vi "ReadInlineCNode.vi"(2 "reference":refnum<vi>) -> (1 "output cluster":T6)   [LabVIEW 2013]
uses:
  <vilib>/Utility/miscctls.llb/LVBoundsTypeDef.ctl
  <vilib>/Utility/miscctls.llb/LVRectTypeDef.ctl
  <vilib>/Utility/miscctls.llb/LVPositionTypeDef.ctl
  <vilib>/Utility/miscctls.llb/LVBreakpointStatusEnum.ctl
  <vilib>/picture/picture.llb/imagedata.ctl
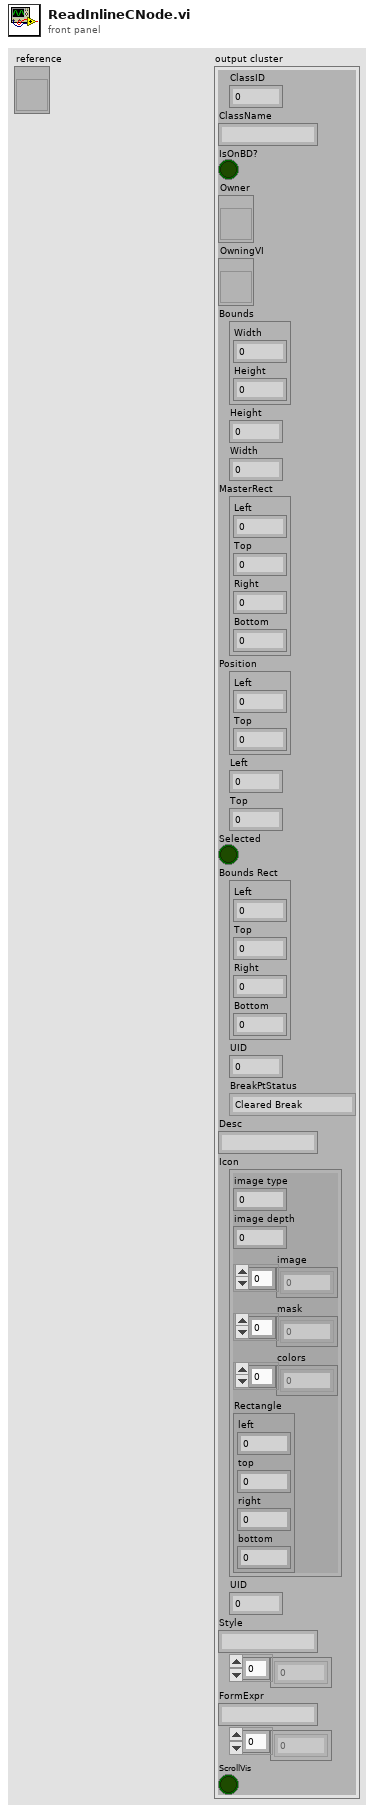
[diagram p1: front panel]
types:
  T1 = typedef "LVBoundsTypeDef.ctl" = cluster{"Width":u32, "Height":u32}
  T2 = typedef "LVRectTypeDef.ctl" = cluster{"Left":i16, "Top":i16, "Right":i16, "Bottom":i16}
  T3 = typedef "LVPositionTypeDef.ctl" = cluster{"Left":i32, "Top":i32}
  T4 = typedef "LVBreakpointStatusEnum.ctl" = enum8{"Cleared Break", "Enabled Break", "Disabled Break"}
  T5 = typedef "imagedata.ctl" = cluster{"image type":i32, "image depth":i32, "image":u8[], "mask":u8[], "colors":u32[], "Rectangle":cluster{"left":i16, "top":i16, "right":i16, "bottom":i16}}
  T6 = cluster{"ClassID":u32, "ClassName":string, "IsOnBD?":bool, "Owner":refnum<vi>, "OwningVI":refnum<vi>, "Bounds":T1, "Height":u32, "Width":u32, "MasterRect":T2, "Position":T3, "Left":i32, "Top":i32, "Selected":bool, "Bounds Rect":T2, "UID":i32, "BreakPtStatus":T4, "Desc":string, "Icon":T5, "UID":i32, "Style":string, i32[], "FormExpr":string, i32[], "ScrollVis":bool}
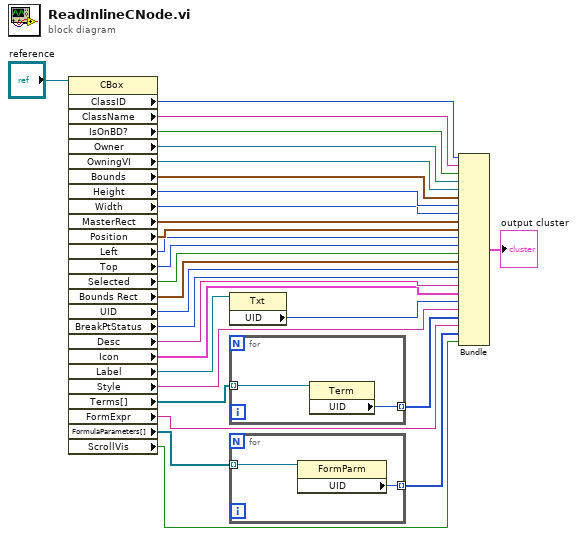
[diagram p0: block diagram]
diagram:
  n1 = property class="CBox"(reference="reference") -> ("ClassID"=w28:u32, "ClassName"=w27:string, "IsOnBD?"=w26:bool, "Owner"=w25:refnum<vi>, "OwningVI"=w24:refnum<vi>, "Bounds"=w23:T1, "Height"=w22:u32, "Width"=w21:u32, "MasterRect"=w20:T2, "Position"=w19:T3, "Left"=w18:i32, "Top"=w17:i32, "Selected"=w16:bool, "Bounds Rect"=w15:T2, "UID"=w14:i32, "BreakPtStatus"=w13:T4, "Desc"=w12:string, "Icon"=w11:T5, "Label"=w10:refnum<vi>, "Style"=w8:string, "Terms[]"=w7:refnum<vi>[], "FormExpr"=w5:string, "FormulaParameters[]"=w4:refnum<vi>[], "ScrollVis"=w2:bool)  [unwired: 1 in, 2 out]
  n2 = property class="Txt"(reference=w10) -> ("UID"=w9:i32)  [unwired: 1 in, 2 out]
  n3 = for {
    tunnel: w7 -> [w31] mode=indexing
    tunnel: [w30] -> w6 mode=indexing
    n4 = property class="Term"(reference=w31) -> ("UID"=w30:i32)  [unwired: 1 in, 2 out]
  }
  n5 = for {
    tunnel: w4 -> [w33] mode=indexing
    tunnel: [w32] -> w3 mode=indexing
    n6 = property class="FormParm"(reference=w33) -> ("UID"=w32:i32)  [unwired: 1 in, 2 out]
  }
  n7 = Bundle("ClassID"=w28, "ClassName"=w27, "IsOnBD?"=w26, "Owner"=w25, "OwningVI"=w24, "Bounds"=w23, "Height"=w22, "Width"=w21, "MasterRect"=w20, "Position"=w19, "Left"=w18, "Top"=w17, "Selected"=w16, "Bounds Rect"=w15, "UID"=w14, "BreakPtStatus"=w13, "Desc"=w12, "Icon"=w11, "UID"=w9, "Style"=w8, w6, "FormExpr"=w5, w3, "ScrollVis"=w2) -> (→"output cluster":T6)  [unwired: 1 in]
